vi "host_remove_white_space.vi"(1 "in":string) -> (0 "out":string)   [LabVIEW 2021]
uses:
  <vilib>/regexp/Match Regular Expression.xnode
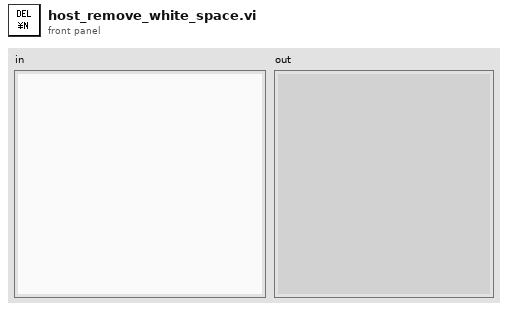
[diagram p1: front panel]
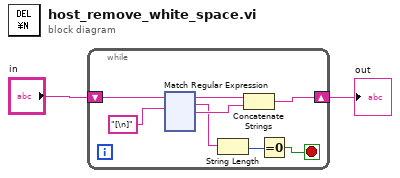
[diagram p0: block diagram]
diagram:
  n1 = while {
    shift-right: [w6] -> w1
    shift-left: "in" -> [w9]
    stop <- w3 stop-if-true
    n2 = xnode "Match Regular Expression"("input string"=w9, "regular expression"="[\n]") -> ("before match"=w8:string, "whole match"=w5:string, "after match"=w7:string)  [unwired: 4 in, 2 out]
    n3 = String Length(string=w5) -> (length=w4:i32)
    n4 = Concatenate Strings(w8, w7) -> (w6:string)
    n5 = Equal To 0?(x=w4) -> (x = 0?=w3:bool)
  }
  "out" <- w1
